vi "MIDI-Console_Entry.vi"(0 "Data In":T1, 11 "Console Entry":string, 13 "Error In":errorcluster) -> (4 "Data Out":T1)   [LabVIEW 2019]
doc: "Adds a new entry to a console log, if an error has occured it will also be logged."
uses:
  Controls/MIDI-Data.ctl
  Controls/MIDI-Message_Array.ctl
  Controls/MIDI-Message_Cluster.ctl
  Controls/Meta_Commands.ctl
  Common/Controls/Application_Message.ctl
  Common/Controls/Application_State.ctl
panel:
  out "Revision Number":u32
  out "Code Size":u32
  out "VI Path":path
  out "VI-filename":string
  out "Timestamp":string
  out "Console log in":string
  out "Console log out":string
  # "VI Input"
  # "VI Output"
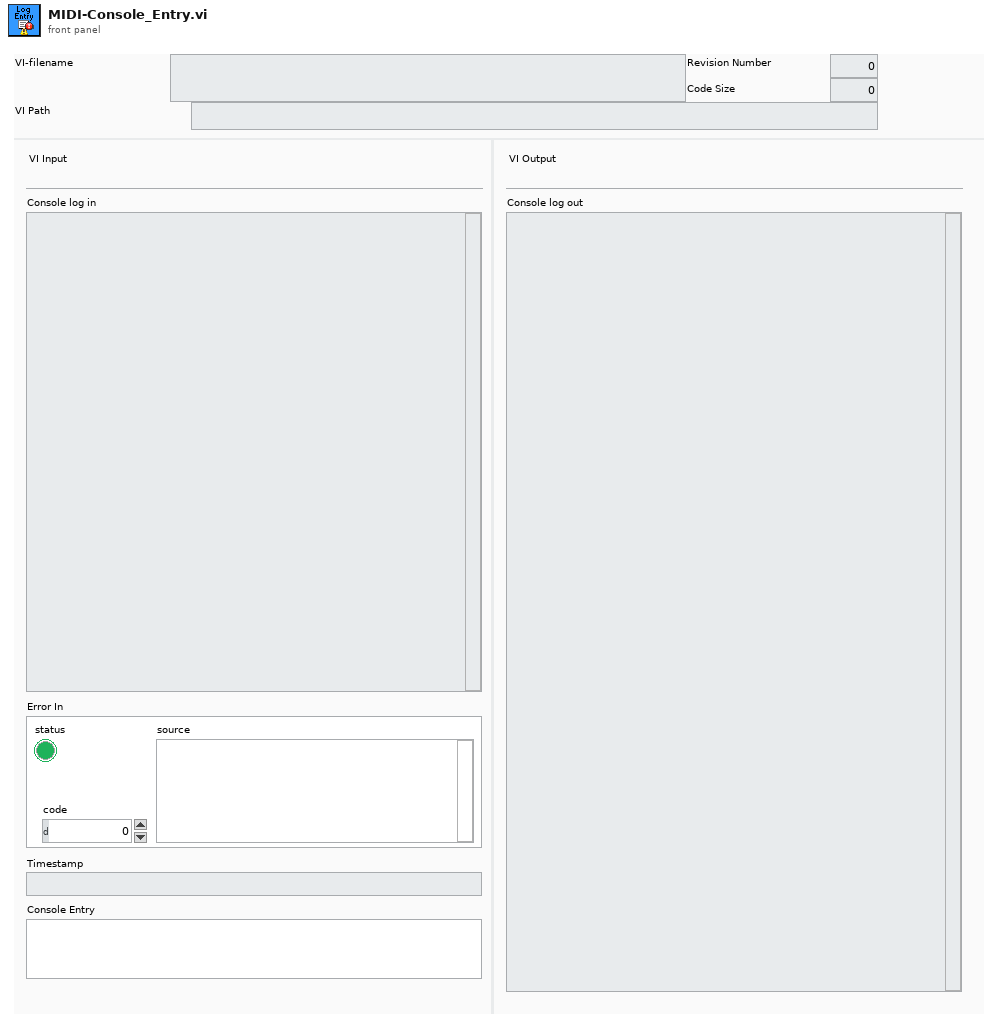
[diagram p1: front panel]
types:
  T1 = typedef "MIDI-Data.ctl" = cluster{"Console log":string, "Payload":variant, "MIDI Message Array":T2, "Timout-Time[ms]":i32, "Queue_MIDI_Handler":refnum<queue>, "To_GUI-Error_message":refnum<user-event>, "To_GUI-msg_list":refnum<user-event>, "CPU(ms)":u32}
  T2 = typedef "MIDI-Message_Array.ctl" = T3[]
  T3 = typedef "MIDI-Message_Cluster.ctl" = cluster{"Message Name":string, "Meta value":i32, "Datastring":string, "Datatype":T4}
  T4 = typedef "Meta_Commands.ctl" = enum16{"No Data", "Pause", "Loop", "Wait for Rx", "Delay", "Break", "MIDI"}
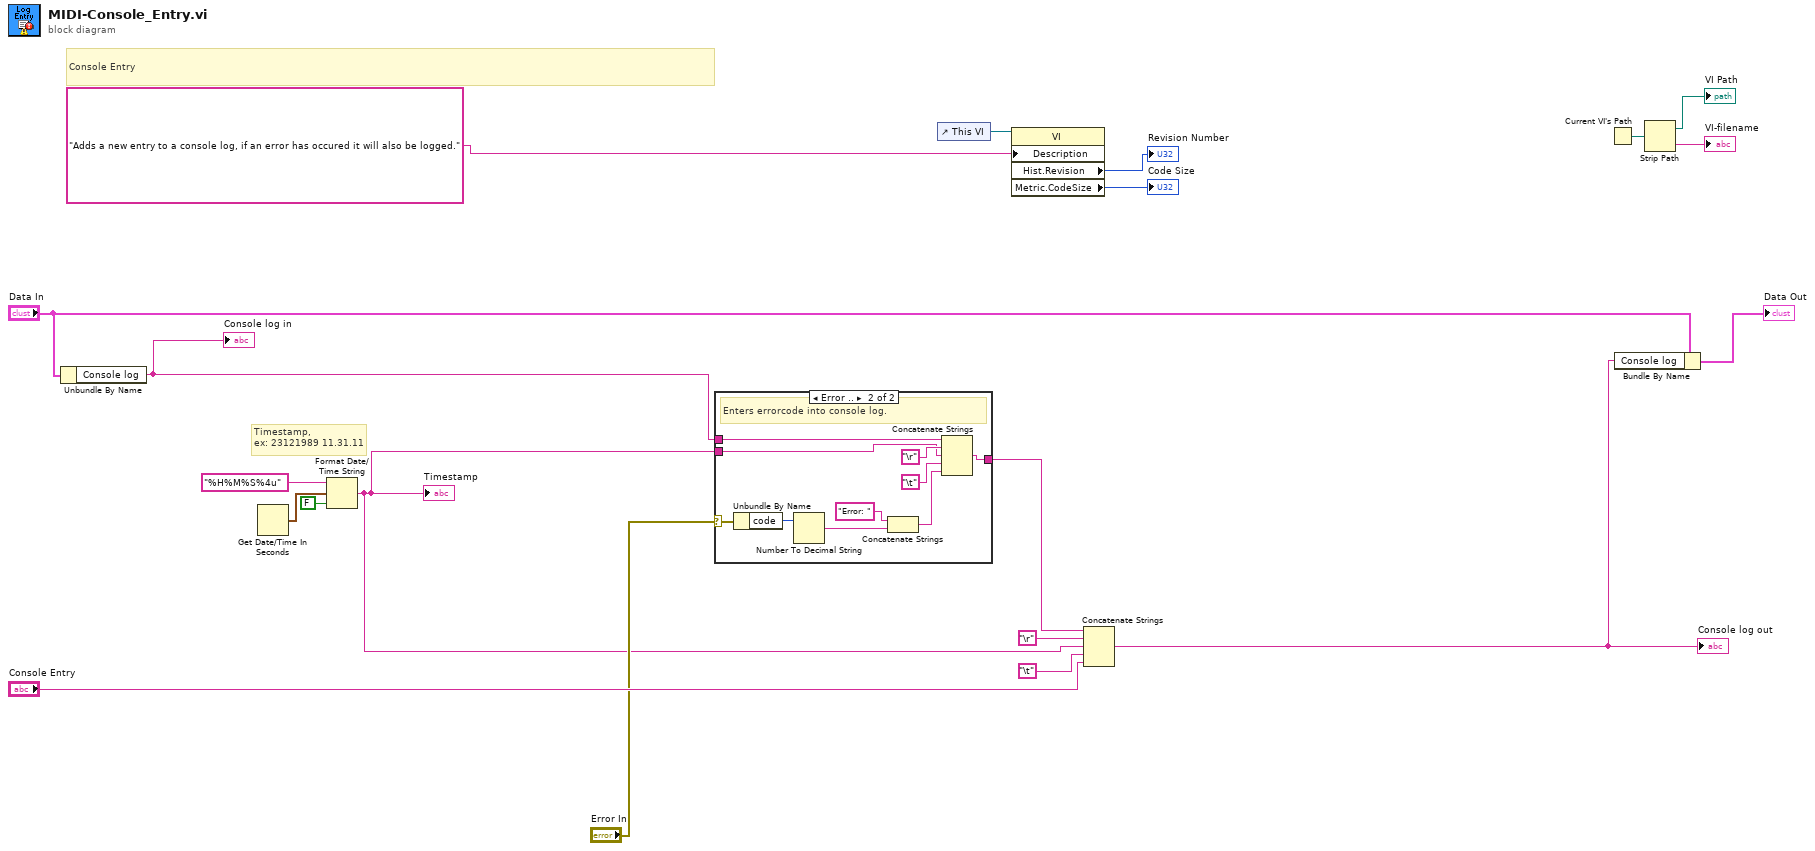
[diagram p0: block diagram]
diagram:
  # "Timestamp, \nex: 23121989 11.31.11"
  # "Console Entry"
  n1 = Unbundle By Name("Data In") -> ("Console log"=w9:string)
  "Console log in" <- w9
  n2 = Get Date/Time In Seconds() -> (seconds since 1Jan1904=w13:timestamp)
  n3 = Format Date/Time String(time format string (%c)="%H%M%S%4u", seconds (now)=w13, UTC format=FALSE) -> (date/time string=w8:string)
  "Timestamp" <- w8
  n4 = case shown="Error .." "Error In" {
    selector: "Error In" -> [_ w23]
    tunnel: w9 -> [w21 w27]
    tunnel: w8 -> [_ w22]
    tunnel: [w21 w24] -> w7
    frame No Error {
    }
    frame Error {
      # "Enters errorcode into console log."
      n5 = Unbundle By Name(w23) -> ("code"=w31:i32)
      n6 = Number To Decimal String(number=w31) -> (decimal integer string=w30:string)  [unwired: 1 in]
      n7 = Concatenate Strings("Error: " ("string"), w30) -> (w29:string)
      n8 = Concatenate Strings(w27, "\r", w22, "\t", w29) -> (w24:string)
    }
  }
  n9 = control-ref of="This VI"() -> (w4:refnum<vi>)
  n10 = property class="VI"(reference=w4, "Description"="Adds a new entry to a console log, if an error has occured it will also be logged.") -> ("Hist.Revision"=→"Revision Number":u32, "Metric.CodeSize"=→"Code Size":u32)  [unwired: 1 in, 2 out]
  n11 = Concatenate Strings(w7, "\r", w8, "\t", "Console Entry") -> (w16:string)
  "Console log out" <- w16
  n12 = Current VI's Path() -> (path=w20:path)
  n13 = Bundle By Name(cluster="Data In", "Console log"=w16) -> (→"Data Out":T1)
  n14 = Strip Path(path=w20) -> (stripped path=→"VI Path":path, name=→"VI-filename":string)
